vi "Acquire Callback.vi"(4 "Cluster":T2, 5 "Event Data":cluster{"sender":refnum<k24>, "e":refnum<k24>}, 6 "Control Ref":refnum<k24>, 7 "Event Common Data":T3) -> ()   [LabVIEW 2019]
uses:
  C:/RM21-MMicrosopeSource/HardwareAdapter/Camera/Dependencies/PVCamNET.dll
  HardwareAdapter/Camera/Dependencies/PVCamNET.dll
  Controls/UIReferenceCtl.ctl
  support/Message Queue/Message Cluster.ctl
  Global.vi
  support/Message Queue/Enqueue Message (Single).vi
  support/Message Queue/Message Queue.lvlib
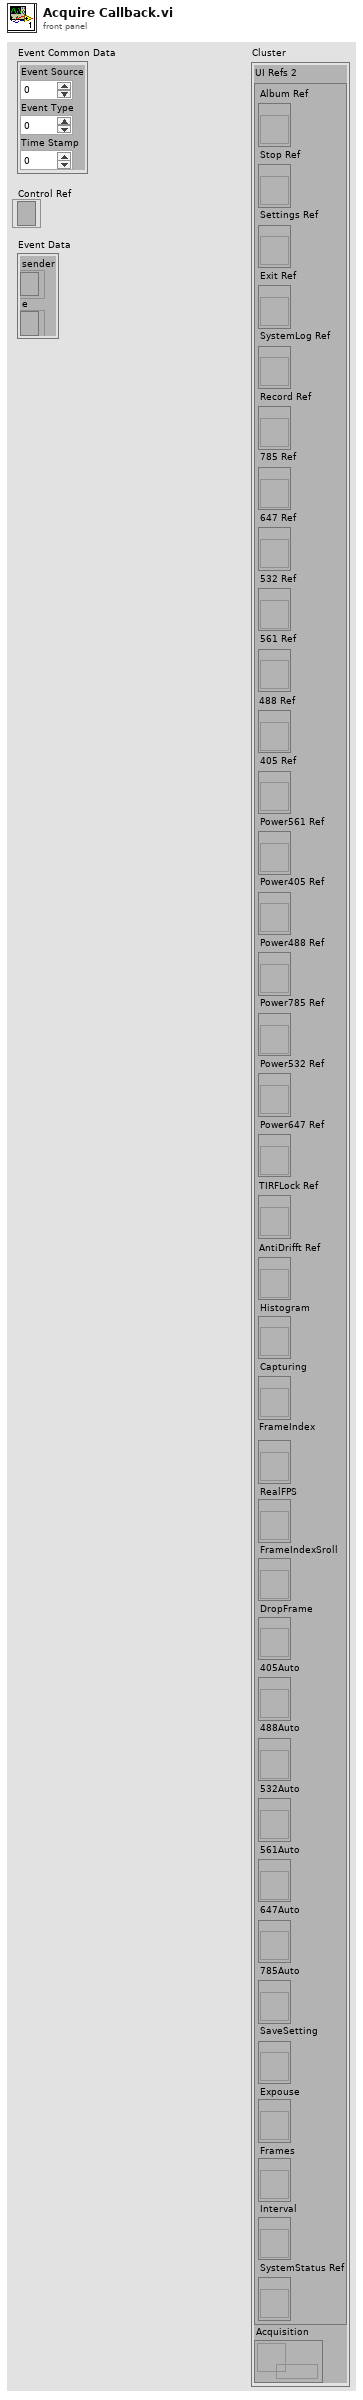
[diagram p1: front panel]
types:
  T1 = typedef "UIReferenceCtl.ctl" = cluster{"Album Ref":refnum<vi>, "Stop Ref":refnum<vi>, "Settings Ref":refnum<vi>, "Exit Ref":refnum<vi>, "SystemLog Ref":refnum<vi>, "Record Ref":refnum<vi>, "785 Ref":refnum<vi>, "647 Ref":refnum<vi>, "532 Ref":refnum<vi>, "561 Ref":refnum<vi>, "488 Ref":refnum<vi>, "405 Ref":refnum<vi>, "Power561 Ref":refnum<vi>, "Power405 Ref":refnum<vi>, "Power488 Ref":refnum<vi>, "Power785 Ref":refnum<vi>, "Power532 Ref":refnum<vi>, "Power647 Ref":refnum<vi>, "TIRFLock Ref":refnum<vi>, "AntiDrifft Ref":refnum<vi>, "Histogram":refnum<vi>, "Capturing":refnum<vi>, "FrameIndex":refnum<vi>, "RealFPS":refnum<vi>, "FrameIndexSroll":refnum<vi>, "DropFrame":refnum<vi>, "405Auto":refnum<vi>, "488Auto":refnum<vi>, "532Auto":refnum<vi>, "561Auto":refnum<vi>, "647Auto":refnum<vi>, "785Auto":refnum<vi>, "SaveSetting":refnum<vi>, "Expouse":refnum<vi>, "Frames":refnum<vi>, "Interval":refnum<vi>, "SystemStatus Ref":refnum<vi>}
  T2 = cluster{"UI Refs 2":T1, "Acquisition":refnum<queue>}
  T3 = cluster{"Event Source":i32, "Event Type":u32, "Time Stamp":u32}
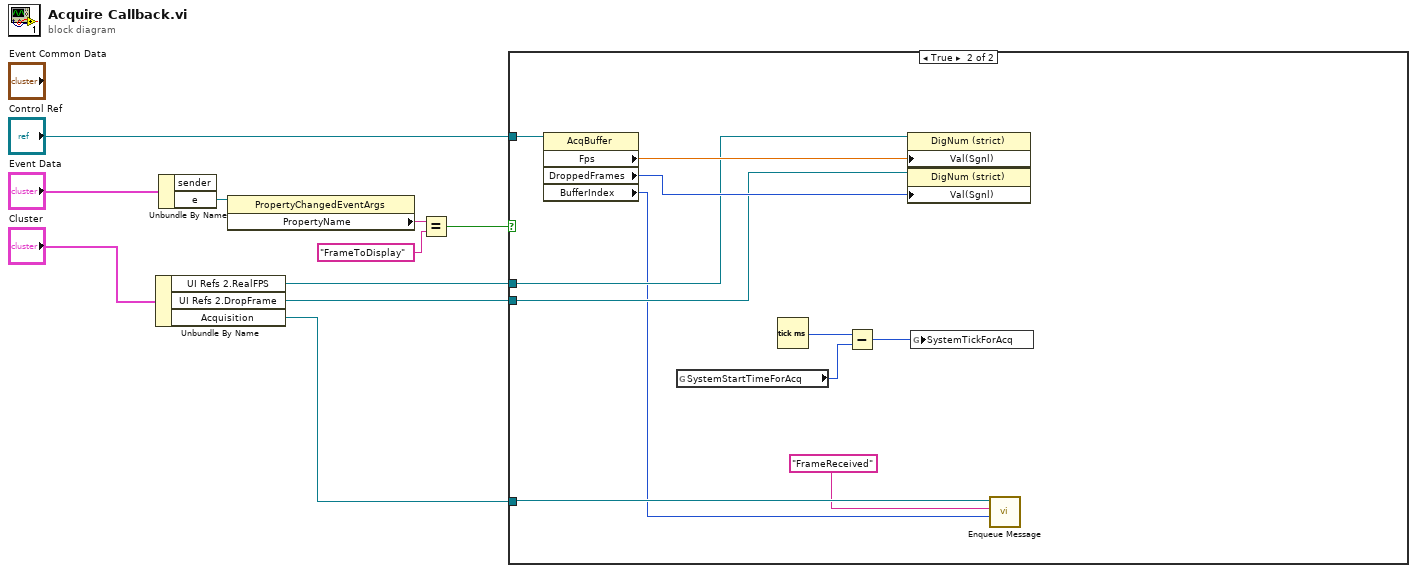
[diagram p0: block diagram]
diagram:
  n1 = Unbundle By Name("Cluster") -> ("UI Refs 2.RealFPS"=w2:refnum<vi>, "UI Refs 2.DropFrame"=w1:refnum<vi>, "Acquisition"=w3:refnum<queue>)
  n2 = Unbundle By Name("Event Data") -> ("e"=w9:refnum<k24>)  [unwired: 1 out]
  n3 = property class="PropertyChangedEventArgs"(reference=w9) -> ("PropertyName"=w8:string)  [unwired: 1 in, 2 out]
  n4 = Equal?(x=w8, y="FrameToDisplay") -> (x = y?=w6:bool)
  n5 = case shown="True" w6 {
    tunnel: "Control Ref" -> [_ w21]
    tunnel: w3 -> [_ w20]
    tunnel: w2 -> [_ w16]
    tunnel: w1 -> [_ w15]
    frame False {
    }
    frame True {
      n6 = property class="AcqBuffer"(reference=w21) -> ("Fps"=w18:sgl, "DroppedFrames"=w17:i32, "BufferIndex"=w14:i32)  [unwired: 1 in, 2 out]
      n7 = global read "Global.vi" "SystemStartTimeForAcq"() -> (w12:u32)
      n8 = Tick Count (ms)() -> (millisecond timer value=w13:u32)
      n9 = Subtract(x=w13, y=w12) -> (x-y=w11:u32)
      n10 = property class="DigNum (strict)"(reference=w16, "Val(Sgnl)"=w18) -> ()  [unwired: 1 in, 2 out]
      n11 = property class="DigNum (strict)"(reference=w15, "Val(Sgnl)"=w17) -> ()  [unwired: 1 in, 2 out]
      n12 = global write "Global.vi" "SystemTickForAcq"(w11) -> ()
      n13 = call-poly "Enqueue Message.vi"("Message Data"=w14, "Message"="FrameReceived", "Message Queue"=w20) -> ()  [unwired: 7 in, 2 out]
    }
  }
